vi "checkFileForChange.vi"(8 "error in (no error)":errorcluster, 11 "AnalysisFile in":refnum<class "AnalysisFile.lvclass">) -> (0 "error out":errorcluster, 3 "AnalysisFile out":refnum<class "AnalysisFile.lvclass">)   [LabVIEW 2009, in "Views.lvlib" / "Camera.lvlib" / "AnalysisFile.lvclass"]
uses:
  AnalysisFile.lvclass
  Tools/Filing/FileNeologist/FileNeologist.lvclass
panel:
  out "x-y":i64
  in  "stop":bool
  out "text":string
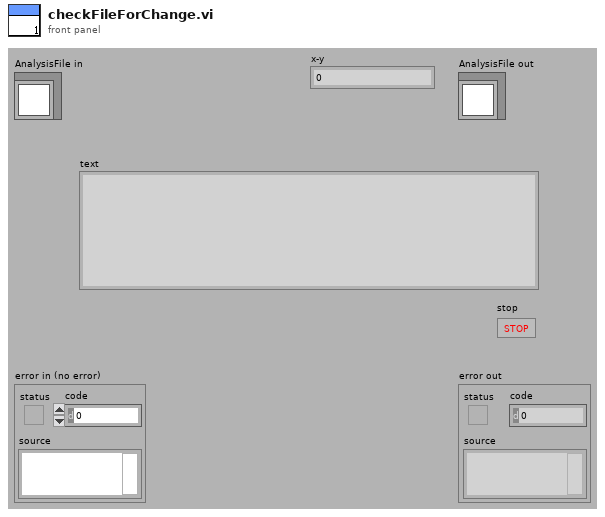
[diagram p1: front panel]
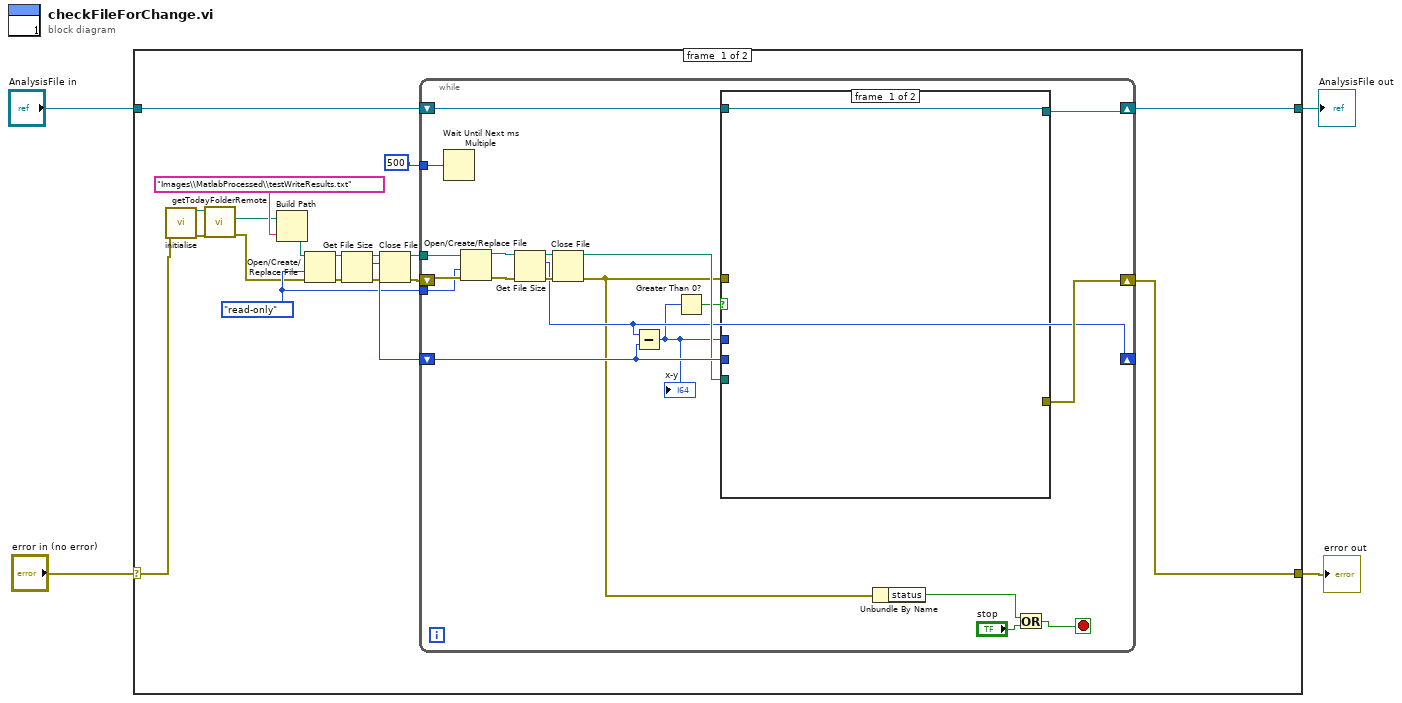
[diagram p0: block diagram]
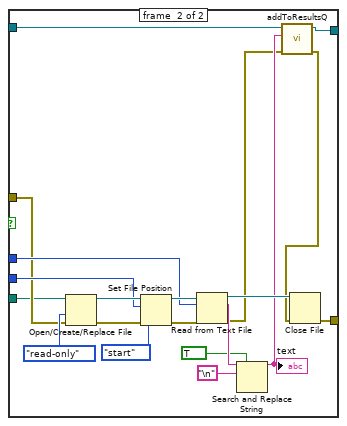
[diagram p2: hidden frame]
diagram:
  n1 = case shown="No Error" "error in (no error)" {
    selector: "error in (no error)" -> [w18 w66]
    tunnel: [w21 w66] -> w3
    tunnel: [w19 w65] -> w1
    tunnel: "AnalysisFile in" -> [w20 w65]
    frame #0 {
      w9 = enum16{"read/write", "read-only", "write-only"}."read-only" ("access (0:read/write)")
      n2 = call "initialise.vi"("error in (no error)"=w18) -> ("error out"=w8:errorcluster, "FileNeologist out"=w7:refnum<class "FileNeologist.lvclass">)  [unwired: 9 in]
      n3 = call "getTodayFolderRemote.vi"("error in (no error)"=w8, "FileNeologist in"=w7) -> ("error out"=w5:errorcluster, "todayFolder"=w6:path)  [unwired: 7 in, 1 out]
      n4 = Build Path(base path=w6, name or relative path="Images\\MatlabProcessed\\testWriteResults.txt") -> (appended path=w16:path)
      n5 = Open/Create/Replace File(file path (use dialog)=w16, error in=w5, access (0:read/write)=w9) -> (refnum out=w15:refnum<file>, error out=w17:errorcluster)  [unwired: 3 in, 1 out]
      n6 = Get File Size(file=w15, error in=w17) -> (refnum out=w13:refnum<file>, size (in bytes)=w11:i64, 0:w14:errorcluster)
      n7 = Close File(refnum=w13, error in=w14) -> (path=w10:path, error out=w12:errorcluster)
      n8 = while {
        tunnel: 500 -> [w43]
        shift-right: [w42] -> w21
        shift-left: w12 -> [w33]
        shift-right: [w31] -> _
        shift-left: w11 -> [w39]
        shift-right: [w40] -> w19
        shift-left: w20 -> [w41]
        tunnel: w10 -> [w34]
        tunnel: w9 -> [w30]
        stop <- w26 stop-if-true
        n9 = Wait Until Next ms Multiple(millisecond multiple=w43) -> ()  [unwired: 1 out]
        n10 = Open/Create/Replace File(file path (use dialog)=w34, error in=w33, access (0:read/write)=w30) -> (refnum out=w37:refnum<file>, error out=w38:errorcluster)  [unwired: 3 in, 1 out]
        n11 = Get File Size(file=w37, error in=w38) -> (refnum out=w35:refnum<file>, size (in bytes)=w31:i64, 0:w36:errorcluster)
        n12 = Close File(refnum=w35, error in=w36) -> (path=w32:path, error out=w25:errorcluster)
        n13 = Subtract(x=w31, y=w39) -> (x-y=w28:i64)
        "x-y" <- w28
        n14 = Greater Than 0?(x=w28) -> (x > 0?=w29:bool)
        n15 = case shown="True" w29 {
          tunnel: w39 -> [_ w60]
          tunnel: w28 -> [_ w57]
          tunnel: [_ w55] -> w42
          tunnel: w41 -> [w44 w51]
          tunnel: [w44 w50] -> w40
          tunnel: w25 -> [_ w46]
          tunnel: w32 -> [_ w45]
          frame #0 {
          }
          frame #1 {
            n16 = Open/Create/Replace File(file path (use dialog)=w45, error in=w46, access (0:read/write)=enum16{"read/write", "read-only", "write-only"}."read-only") -> (refnum out=w63:refnum<file>, error out=w62:errorcluster)  [unwired: 3 in, 1 out]
            n17 = Set File Position(offset (in bytes) (0)=w60, refnum=w63, from (0:start)=enum16{"start", "end", "current"}."start", error in=w62) -> (refnum out=w58:refnum<file>, error out=w59:errorcluster)
            n18 = Read from Text File(file (use dialog)=w58, count=w57, error in=w59) -> (refnum out=w56:refnum<file>, text=w54:string, error out=w48:errorcluster)  [unwired: 1 in, 1 out]
            n19 = Search and Replace String(replace all?=TRUE ("replace all? (F)"), input string=w54, search string="\n") -> (result string=w49:string)  [unwired: 5 in, 3 out]
            "text" <- w49
            n20 = call "addToResultsQ.vi"("error in (no error)"=w48, "Results"=w49, "AnalysisFile in"=w51) -> ("error out"=w47:errorcluster, "AnalysisFile out"=w50:refnum<class "AnalysisFile.lvclass">)  [unwired: 7 in]
            n21 = Close File(refnum=w56, error in=w47) -> (error out=w55:errorcluster)  [unwired: 1 out]
          }
        }
        n22 = Unbundle By Name(w25) -> ("status"=w24:bool)
        n23 = Or(x=w24, y="stop") -> (x .or. y?=w26:bool)
      }
    }
    frame #1 {
    }
  }
  "error out" <- w3
  "AnalysisFile out" <- w1
